vi "PPS_TRAJ_Creation_AbsSwerve-2.vi"(8 "End Pose  ENG":T6={"TRANSLATION"={"X"=0.0, "Y"=0.0}, "ROTATION"={"VALUE"=0.0, "COS"=1.0, "SIN"=0.0}} {"ROTATION"."SIN" format="%13.4f"; "ROTATION"."COS" format="%13.4f"; "ROTATION"."VALUE" format="%13.4f"; "TRANSLATION"."Y" format="%14.3f"; "TRANSLATION"."X" format="%14.3f"}, 9 "Current Pose SI":T6={"TRANSLATION"={"X"=0.0, "Y"=0.0}, "ROTATION"={"VALUE"=0.0, "COS"=1.0, "SIN"=0.0}} {"ROTATION"."SIN" format="%13.4f"; "ROTATION"."COS" format="%13.4f"; "ROTATION"."VALUE" format="%13.4f"; "TRANSLATION"."Y" format="%14.3f"; "TRANSLATION"."X" format="%14.3f"}, 10 "Max Velocity M/S":dbl=3.2 format="%17.3f", 11 "SWERVE_DRIVE_KINEMATICS":T1 {"SavedModuleStates"."Angle"."SIN" format="%13.4f"; "SavedModuleStates"."Angle"."COS" format="%13.4f"; "SavedModuleStates"."Angle"."VALUE" format="%13.4f"; "PrevCoR"."Y" format="%14.3f"; "PrevCoR"."X" format="%14.3f"; "Modules"."Y" format="%14.3f"; "Modules"."X" format="%14.3f"}) -> (0 "Path\nCreation\nError":bool, 1 "PathPlannerTrajectory":T7 {"States"."TargetHolonomicRotation"."SIN" format="%13.4f"; "States"."TargetHolonomicRotation"."COS" format="%13.4f"; "States"."TargetHolonomicRotation"."VALUE" format="%13.4f"; "States"."Heading"."SIN" format="%13.4f"; "States"."Heading"."COS" format="%13.4f"; "States"."Heading"."VALUE" format="%13.4f"; "States"."PositionMeters"."Y" format="%14.3f"; "States"."PositionMeters"."X" format="%14.3f"}, 3 "TotalTImeSecs":dbl)   [LabVIEW 2019]
uses:
  <vilib>/Rock Robotics/WPI/ThirdParty/MJansen/PathPlanner/TypeDef/PathPlannerTrajectory.ctl
  <vilib>/Rock Robotics/WPI/ThirdParty/MJansen/PathPlanner/TypeDef/PathPlannerTrajectoryState.ctl
  <vilib>/Rock Robotics/WPI/ThirdParty/JAS_Junk/TrajLib/TypeDef/TRANSLATION2D.ctl
  <vilib>/Rock Robotics/WPI/ThirdParty/JAS_Junk/TrajLib/TypeDef/ROTATION2D.ctl
  <vilib>/Rock Robotics/WPI/ThirdParty/MJansen/PathPlanner/TypeDef/PathPlannerPathConstraints.ctl
  <vilib>/Rock Robotics/WPI/ThirdParty/JAS_Junk/TrajLib/TypeDef/POSE2D.ctl
  <vilib>/Rock Robotics/WPI/ThirdParty/JAS_Junk/TrajLib/TypeDef/SWERVE_DRIVE_KINEMATICS.ctl
  <vilib>/Analysis/Matrix/Datatypes/RealMatrix.ctl
  <vilib>/Rock Robotics/WPI/ThirdParty/JAS_Junk/TrajLib/TypeDef/SWERVE_DRIVE_MODULE_STATE.ctl
  <vilib>/Rock Robotics/WPI/ThirdParty/JAS_Junk/TrajLib/Util_CalcDist.vi
  <vilib>/Rock Robotics/WPI/ThirdParty/JAS_Junk/TrajLib/Rotation2d_CreateXY.vi
  <vilib>/Rock Robotics/WPI/ThirdParty/JAS_Junk/TrajLib/Rotation2d_CreateAngle.vi
  <vilib>/Rock Robotics/WPI/ThirdParty/JAS_Junk/TrajLib/Pose2d_getTranslation.vi
  <vilib>/Rock Robotics/WPI/ThirdParty/JAS_Junk/TrajLib/Pose2d_getRotation.vi
  <vilib>/Rock Robotics/WPI/ThirdParty/JAS_Junk/TrajLib/Translation2d_Create_DistAng.vi
  <vilib>/Rock Robotics/WPI/ThirdParty/JAS_Junk/TrajLib/Rotation2d_Plus.vi
  <vilib>/Rock Robotics/WPI/ThirdParty/JAS_Junk/TrajLib/Rotation2d_CreateAngleDegrees.vi
  <vilib>/Rock Robotics/WPI/ThirdParty/JAS_Junk/TrajLib/Rotation2d_GetAngleCosSin.vi
  <vilib>/Rock Robotics/WPI/ThirdParty/JAS_Junk/TrajLib/Rotation2d_RotateBy.vi
  <vilib>/Rock Robotics/WPI/ThirdParty/JAS_Junk/TrajLib/Conv_Deg_Radians.vi
  <vilib>/Rock Robotics/WPI/ThirdParty/MJansen/PathPlanner/PathPlanner24.lvlib
  <vilib>/Rock Robotics/WPI/ThirdParty/JAS_Junk/TrajLib/Trajectory_Library.lvlib
  <vilib>/Analysis/Matrix/NI_Matrix.lvlib
panel:
  in  "End Velocity M/S":dbl format="%#_13g"
  in  "Start Angual Vel Rad/S":dbl format="%#_13g"
  in  "Start Y Vel M/S":dbl format="%#_13g"
  in  "Start X Vel M/S":dbl format="%#_13g"
  in  "MaxAngularAccel Radians.Sec^2":dbl=2.4 format="%17.3f"
  out "Trajectory":cluster{dbl[], dbl[]}(graph)
  out "Trajectory State\nCount":i32
  in  "MaxAcceleration M/S^2":dbl=2.8 format="%17.1f"
  in  "MaxAngularVel  Radians/Sec":dbl=1.8 format="%17.3f"
  # "Create PathPlanner Path/Trajectory Sample"
  # "This VI is designed to be called by BEGIN.VI, but can be executed directly to test trajectory parameters."
  # "CREATED TRAJECTORY INFORMATION"
  # "PATH CONFIGURATION"
  # "PATH DEFINITION"
  # "There can be as many points as needed."
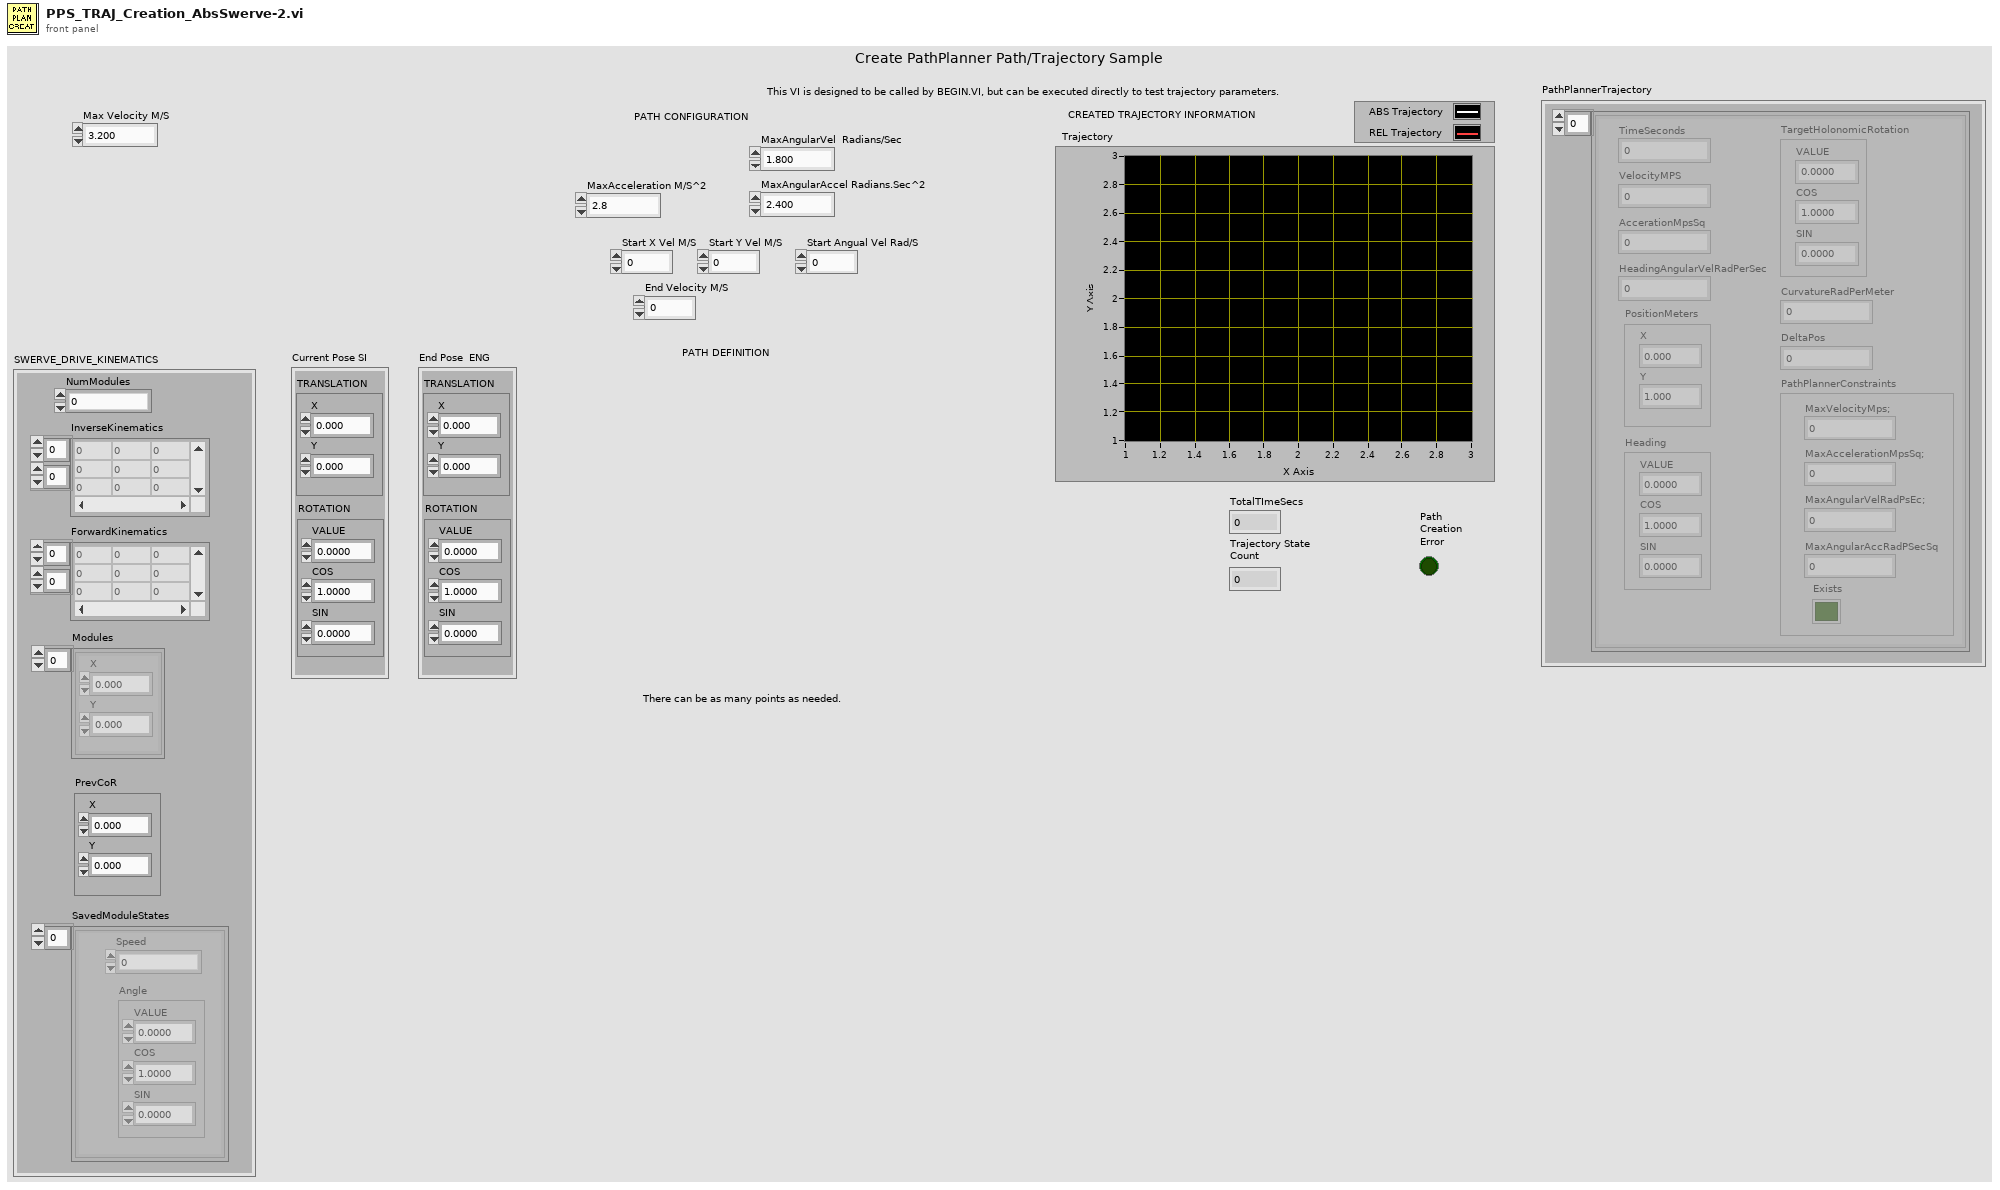
[diagram p1: front panel]
types:
  T1 = typedef "Trajectory_Library.lvlib/SWERVE_DRIVE_KINEMATICS.ctl" = cluster{"NumModules":i32, "InverseKinematics":T2, "ForwardKinematics":T2, "Modules":T3[], "PrevCoR":T3, "SavedModuleStates":T4[]}
  T2 = typedef "NI_Matrix.lvlib/RealMatrix.ctl" = dbl[][]
  T3 = typedef "Trajectory_Library.lvlib/TRANSLATION2D.ctl" = cluster{"X":dbl, "Y":dbl}
  T4 = typedef "Trajectory_Library.lvlib/SWERVE_DRIVE_MODULE_STATE.ctl" = cluster{"Speed":dbl, "Angle":T5}
  T5 = typedef "Trajectory_Library.lvlib/ROTATION2D.ctl" = cluster{"VALUE":dbl, "COS":dbl, "SIN":dbl}
  T6 = typedef "Trajectory_Library.lvlib/POSE2D.ctl" = cluster{"TRANSLATION":T3, "ROTATION":T5}
  T7 = typedef "PathPlanner24.lvlib/PathPlannerTrajectory.ctl" = cluster{"States":T8[]}
  T8 = typedef "PathPlanner24.lvlib/PathPlannerTrajectoryState.ctl" = cluster{"TimeSeconds":dbl, "VelocityMPS":dbl, "AccerationMpsSq":dbl, "HeadingAngularVelRadPerSec":dbl, "PositionMeters":T3, "Heading":T5, "TargetHolonomicRotation":T5, "CurvatureRadPerMeter":dbl, "PathPlannerConstraints":T9, "DeltaPos":dbl}
  T9 = typedef "PathPlanner24.lvlib/PathPlannerPathConstraints.ctl" = cluster{"MaxVelocityMps;":dbl, "MaxAccelerationMpsSq;":dbl, "MaxAngularVelRadPsEc;":dbl, "MaxAngularAccRadPSecSq":dbl, "Exists":bool}
  T10 = typedef "PathPlanner24.lvlib/PathPlannerRotationTarget.ctl" = cluster{"target":T5, "WaypointRelativePosition":dbl, "Exists":bool}
  T11 = typedef "Trajectory_Library.lvlib/CHASSIS_SPEEDS.ctl" = cluster{"vX":dbl, "vY":dbl, "vOmega":dbl}
  T12 = typedef "PathPlanner24.lvlib/PathPlannerGoalEndState.ctl" = cluster{"Velocity":dbl, "Rotation":T5}
  T13 = typedef "PathPlanner24.lvlib/PathPlannerPath.ctl" = cluster{"BezierPoints":T3[], "PreviewStartingRotation":T5, "Reversed":bool, "RotationTargets":T10[], "ConstraintZones":T14[], "EventMarkers":T15[], "GlobalConstraints":T9, "GoalEndState":T12, "AllPoints":T18[]}
  T14 = typedef "PathPlanner24.lvlib/PathPlannerConstraintsZone.ctl" = cluster{"minWaypointPos":dbl, "maxWaypointPos":dbl, "Constraints":T9, "Present":bool}
  T15 = typedef "PathPlanner24.lvlib/PathPlannerEventMarker.ctl" = cluster{"WaypointRelativePos":dbl, "minimumTriggerDistance":dbl, "markerPos":T3, "lastRobotPos":T3, "Command":T16, "markerPos Exists":bool, "LastRobotPoseExists":bool}
  T16 = typedef "PathPlanner24.lvlib/PathPlannerCommandUtil.ctl" = cluster{"waitTime":dbl, "name":string, "pathName":string, "commands":cluster{"type":string, "waitTime":dbl, "name":string, "pathName":string}[], "type":T17}
  T17 = typedef "PathPlanner24.lvlib/PathPlanner_CommandUtilType_ENUM.ctl" = enum16{"Unknown", "Wait", "Named", "Path", "Sequential", "Parallel", "Race", "Deadline"}
  T18 = typedef "PathPlanner24.lvlib/PathPlannerPathPoint.ctl" = cluster{"Position":T3, "HolonomicRotation":T5, "DistAlongPath":dbl, "CurveRadius":dbl, "MaxV":dbl, "Constraints":T9, "HolonomicRotationExists":bool}
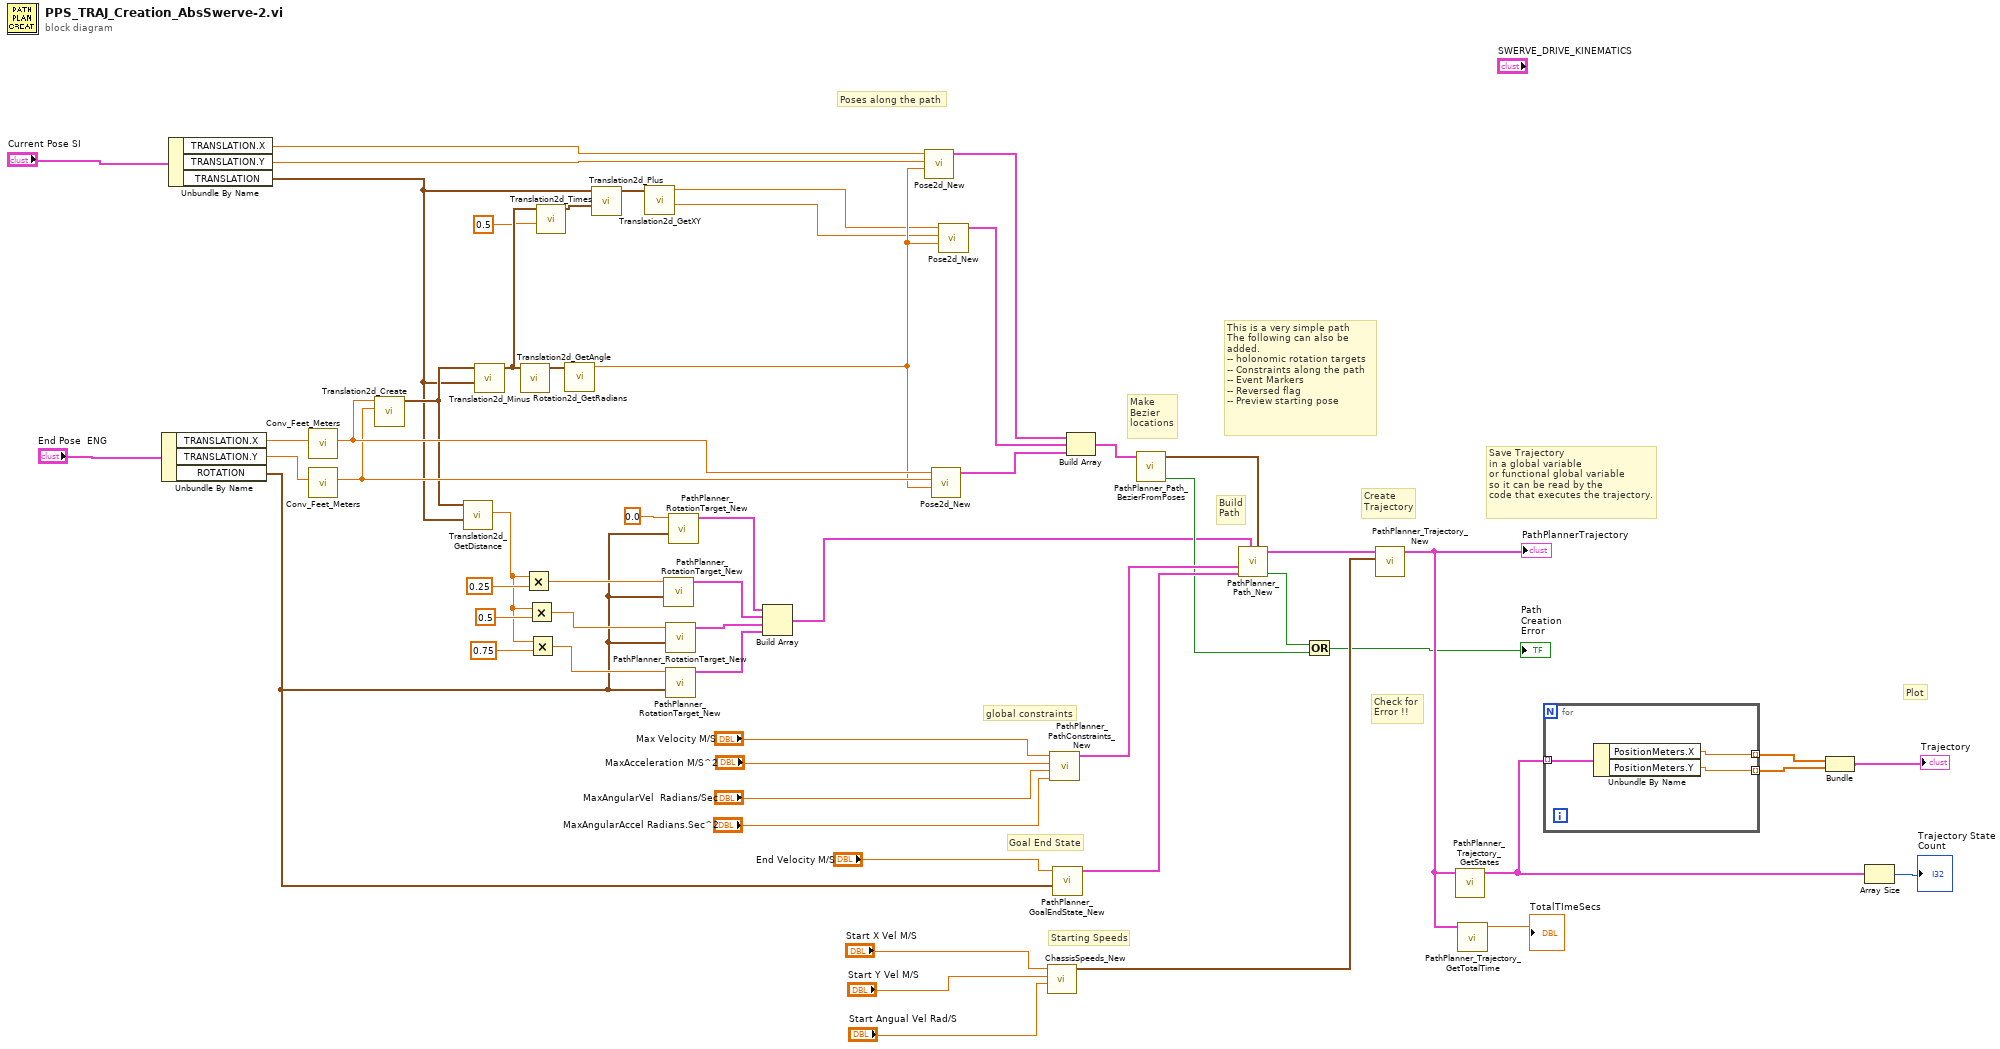
[diagram p0: block diagram]
diagram:
  # "This is a very simple path\nThe following can also be\nadded.\n-- holonomic rotation targets\n-- Constraints along the path\n-- Event Markers\n-- Reversed flag\n-- Preview starting pose"
  # "Plot"
  # "Save Trajectory\nin a global variable\nor functional global variable\nso it can be read by the \ncode that executes the trajectory."
  # "Create\nTrajectory"
  # "Check for\nError !!"
  # "Starting Speeds"
  # "Goal End State"
  # "global constraints"
  # "Make\nBezier\nlocations"
  # "Build\nPath"
  # "Poses along the path"
  n1 = Unbundle By Name("End Pose  ENG") -> ("TRANSLATION.X"=w37:dbl, "TRANSLATION.Y"=w36:dbl, "ROTATION"=w4:T5)
  n2 = Unbundle By Name("Current Pose SI") -> ("TRANSLATION.X"=w32:dbl, "TRANSLATION.Y"=w31:dbl, "TRANSLATION"=w17:T3)
  n3 = call <vilib>:"Conv_Feet_Meters.vi"("Feet"=w37) -> ("Meters"=w30:dbl)  [unwired: 10 in]
  n4 = call <vilib>:"Conv_Feet_Meters.vi"("Feet"=w36) -> ("Meters"=w29:dbl)  [unwired: 10 in]
  n5 = call <vilib>:"Translation2d_Create.vi"("Y"=w29, "X"=w30) -> ("TRANSLATION"=w20:T3)  [unwired: 9 in]
  n6 = call <vilib>:"Translation2d_GetDistance.vi"("other Translation"=w17, "In Translation"=w20) -> ("Distance"=w7:dbl)  [unwired: 9 in]
  n7 = call <vilib>:"Translation2d_Minus.vi"("other Translation"=w17, "In Translation"=w20) -> ("Out Translation"=w19:T3)  [unwired: 9 in]
  n8 = call <vilib>:"Translation2d_GetAngle.vi"("In Translation"=w19) -> ("Angle_Rotation2d"=w35:T5)  [unwired: 10 in]
  n9 = Multiply(x=w7, y=0.25) -> (x*y=w21:dbl)
  n10 = Multiply(x=w7, y=0.5) -> (x*y=w6:dbl)
  n11 = Multiply(x=w7, y=0.75) -> (x*y=w5:dbl)
  n12 = call <vilib>:"Translation2d_Times.vi"("Scalar"=0.5, "In Translation"=w19) -> ("Out Translation"=w16:T3)  [unwired: 9 in]
  n13 = call <vilib>:"Rotation2d_GetRadians.vi"("in ROTATION"=w35) -> ("AngleRadians"=w12:dbl)  [unwired: 10 in]
  n14 = call <vilib>:"Translation2d_Plus.vi"("other Translation"=w16, "In Translation"=w17) -> ("Out Translation"=w13:T3)  [unwired: 9 in]
  n15 = call <vilib>:"Translation2d_GetXY.vi"("In Translation"=w13) -> ("Y"=w10:dbl, "X"=w11:dbl)  [unwired: 9 in]
  n16 = call <vilib>:"PathPlanner_RotationTarget_New.vi"("target"=w4, "WaypointRelativePosition"=w21) -> ("RotationTarget"=w3:T10)  [unwired: 9 in]
  n17 = call <vilib>:"PathPlanner_RotationTarget_New.vi"("target"=w4, "WaypointRelativePosition"=w6) -> ("RotationTarget"=w2:T10)  [unwired: 9 in]
  n18 = call <vilib>:"PathPlanner_RotationTarget_New.vi"("target"=w4, "WaypointRelativePosition"=w5) -> ("RotationTarget"=w1:T10)  [unwired: 9 in]
  n19 = call <vilib>:"PathPlanner_RotationTarget_New.vi"("target"=w4, "WaypointRelativePosition"=0.0) -> ("RotationTarget"=w24:T10)  [unwired: 9 in]
  n20 = Build Array(w24, w3, w2, w1) -> (w23:T10[])
  n21 = call <vilib>:"Pose2d_New.vi"("Heading"=w12, "Y"=w31, "X"=w32) -> ("out POSe"=w15:T6)  [unwired: 8 in]
  n22 = call <vilib>:"Pose2d_New.vi"("Heading"=w12, "Y"=w29, "X"=w30) -> ("out POSe"=w49:T6)  [unwired: 8 in]
  n23 = call <vilib>:"Pose2d_New.vi"("Heading"=w12, "Y"=w10, "X"=w11) -> ("out POSe"=w14:T6)  [unwired: 8 in]
  n24 = call <vilib>:"ChassisSpeeds_New.vi"("vAngular"="Start Angual Vel Rad/S", "vY"="Start Y Vel M/S", "vX"="Start X Vel M/S") -> ("CHASSIS"=w58:T11)  [unwired: 8 in]
  n25 = call <vilib>:"PathPlanner_PathConstraints_New.vi"("MaxAngularAccRadPSecSq"="MaxAngularAccel Radians.Sec^2", "MaxAngularVelRadPsEc;"="MaxAngularVel  Radians/Sec", "MaxAccelerationMpsSq;"="MaxAcceleration M/S^2", "MaxVelocityMps;"="Max Velocity M/S") -> ("PathPlannerConstraints"=w51:T9)  [unwired: 7 in]
  n26 = call <vilib>:"PathPlanner_GoalEndState_New.vi"("Rotation"=w4, "Velocity"="End Velocity M/S") -> ("GoalEndState"=w53:T12)  [unwired: 9 in]
  n27 = Build Array(w15, w14, w49) -> (w48:T6[])
  n28 = call <vilib>:"PathPlanner_Path_BezierFromPoses.vi"("Poses"=w48) -> ("Error"=w26:bool, "Bezier"=w50:T3[])  [unwired: 9 in]
  n29 = call <vilib>:"PathPlanner_Path_New.vi"("BezierPoints"=w50, "HolonomicRotations"=w23, "GoalEndState"=w53, "GlobalConstraints"=w51) -> ("Error"=w27:bool, "PathPlannerPath"=w54:T13)  [unwired: 6 in]
  n30 = Or(x=w27, y=w26) -> (x .or. y?=→"Path\nCreation\nError":bool)
  n31 = call <vilib>:"PathPlanner_Trajectory_New.vi"("StartingSpeeds"=w58, "Path"=w54) -> ("PathPlannerTrajectory"=w43:T7)  [unwired: 9 in]
  "PathPlannerTrajectory" <- w43
  n32 = call <vilib>:"PathPlanner_Trajectory_GetStates.vi"("PathPlannerTrajectory"=w43) -> ("PathPlannerStates"=w44:T8[])  [unwired: 10 in]
  n33 = call <vilib>:"PathPlanner_Trajectory_GetTotalTime.vi"("PathPlannerTrajectory"=w43) -> ("TotalTimeSeconds"=→"TotalTImeSecs":dbl)  [unwired: 10 in]
  n34 = for {
    tunnel: [w62] -> w46 mode=indexing
    tunnel: [w61] -> w47 mode=indexing
    tunnel: w44 -> [w60] mode=indexing
    n35 = Unbundle By Name(w60) -> ("PositionMeters.X"=w62:dbl, "PositionMeters.Y"=w61:dbl)
  }
  n36 = Bundle(w46, w47) -> (→"Trajectory":cluster{dbl[], dbl[]})  [unwired: 1 in]
  n37 = Array Size(array=w44) -> (size(s)=→"Trajectory State\nCount":i32)
